vi "JKISM++ Status Change Event.vi"(8 "Error in":errorcluster caption="Error in (no error)", 11 "Name(\"\" to use uuid) in":string) -> (0 "Error out":errorcluster, 3 "Status Change Event":refnum<user-event>)   [LabVIEW 2014, in "JKI State Machine++.lvlib"]
doc: "Obtain JKISM++ Global Log Event Reference.\n\n<b>Inputs:</b>\n - <b>Error in</b>: Error cluster\n\n<b>Outputs:</b>\n - <b>JKISM Global Log Event</b>: User event reference for JKISM global log.\n - <b>Error out</b>: Error cluster"
uses:
  JKI State Machine++.lvlib
  _Support/Typedef/_JKISM Status Change Event Data.ctl
  _Support/JKISMQ/_JKISMQFGVOPER.ctl
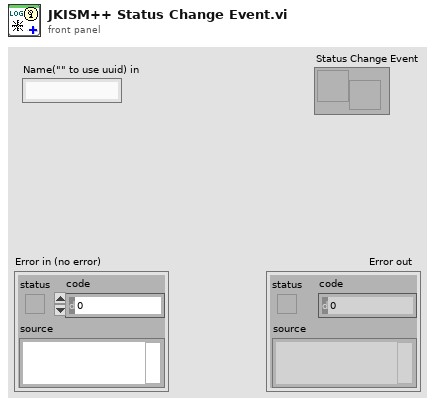
[diagram p1: front panel]
types:
  T1 = typedef "JKI State Machine++.lvlib/_JKISMQFGVOPER.ctl" = enum16{"Get By Name", "List", "Check If Name Exists", "Release", "Module Status", "Create Status Event Handler", "Destroy Status Event Handler"}
  T2 = typedef "JKI State Machine++.lvlib/_JKISMQ.ctl" = cluster{"Module Name":string, "Queue":refnum<queue>, "Locked Status":refnum<data-value>, "Mode":T3, "User Event":refnum<user-event>, "Queue Count":i32, "Status Change Event":refnum<user-event>}
  T3 = typedef "JKI State Machine++.lvlib/_JKISM_MODE.ctl" = enum16{"Stand Alone", "JKISM", "Action Worker"}
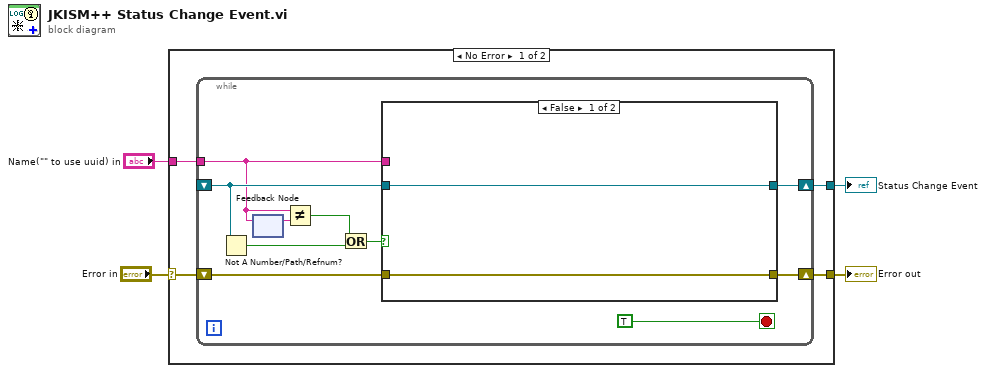
[diagram p0: block diagram]
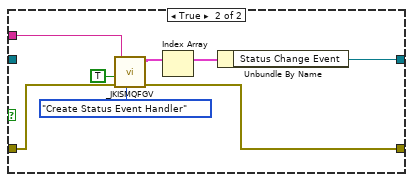
[diagram p2: hidden frame]
diagram:
  n1 = case shown="No Error" "Error in" {
    selector: "Error in" -> [w7 w29]
    tunnel: [w8 _] -> w2
    tunnel: [w6 w29] -> w3
    tunnel: "Name(\"\" to use uuid) in" -> [w5 _]
    frame No Error {
      n2 = while {
        shift-right: [w16] -> w6
        shift-left: w7 -> [w17]
        shift-right: [w18] -> w8
        shift-left: _ -> [w14]
        tunnel: w5 -> [w12]
        stop <- TRUE stop-if-true
        n3 = Not A Number/Path/Refnum?(number/path/refnum=w14) -> (NaN/Path/Refnum?=w10:bool)
        n4 = feedback-in #1(w12) -> ()
        n5 = feedback #1() -> (w11:string)  [unwired: 1 in]
        n6 = Not Equal?(x=w12, y=w11) -> (x != y?=w9:bool)
        n7 = Or(x=w9, y=w10) -> (x .or. y?=w13:bool)
        n8 = case shown="False" w13 {
          tunnel: [w20 w23] -> w18
          tunnel: w17 -> [w19 w26]
          tunnel: [w19 w27] -> w16
          tunnel: w14 -> [w20 _]
          tunnel: w12 -> [_ w22]
          frame False {
          }
          frame True {
            n9 = call "_JKISMQFGV.vi"("Operation"=_JKISMQFGVOPER."Create Status Event Handler", "Error in"=w26, "create if not found? (T)"=TRUE, "Name(\"\" to use uuid) in"=w22) -> ("Error out"=w27:errorcluster, "Array"=w25:T2[])  [unwired: 4 in, 2 out]
            n10 = Index Array(array=w25) -> (element=w24:T2)  [unwired: 1 in]
            n11 = Unbundle By Name(w24) -> ("Status Change Event"=w23:refnum<user-event>)
          }
        }
      }
    }
    frame Error {
    }
  }
  "Error out" <- w3
  "Status Change Event" <- w2
